vi "FTP_Event.vi"(11 "Event":refnum<user-event>) -> ()   [LabVIEW 2013]
uses:
  Ctrls/CallbackEvent.ctl
  Ctrls/Action.ctl
  edtFTPnet.lvlib
panel:
  in  "Event 2":T1={"Action"=enum."<None>", "Direction"=1, "LocalFilePath"="", "RemoteFilename"=""} {"Direction" items=["UPLOAD"=1, "DOWNLOAD"=2]}
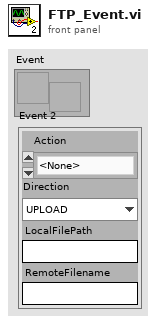
[diagram p1: front panel]
types:
  T1 = typedef "edtFTPnet.lvlib/CallbackEvent.ctl" = cluster{"Action":T2, "Direction":i32, "LocalFilePath":string, "RemoteFilename":string}
  T2 = typedef "Action.ctl" = enum16{"<None>", "TransferStarted", "Transfering", "TransferCompleted"}
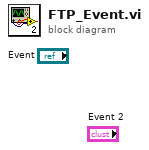
[diagram p0: block diagram]
diagram:
